vi "StopPull.vi"() -> ()   [LabVIEW 2009]
uses:
  <instrlib>/Newport ESP301/Newport ESP301.lvlib
panel:
  in  "Feedback Filter Settings":T1
  in  "Master Axis":i32
  out "error out":errorcluster
  in  "error in":errorcluster
  out "VISA resource name out":refnum<visa-resource-name>
  in  "VISA resource name":refnum<visa-resource-name>
  in  "Slave Axis":i32
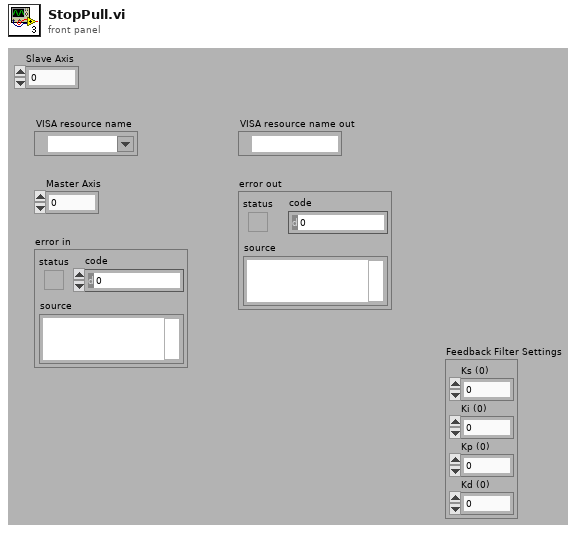
[diagram p1: front panel]
types:
  T1 = cluster{"Ks (0)":dbl, "Ki (0)":dbl, "Kp (0)":dbl, "Kd (0)":dbl}
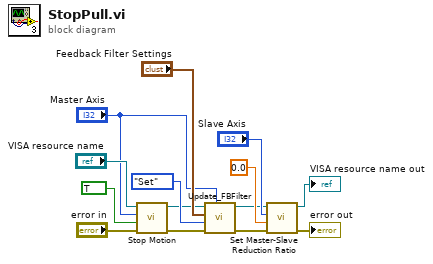
[diagram p0: block diagram]
diagram:
  n1 = call <instrlib>:"Stop Motion.vi"("error in (no error)"="error in", "Stop all axes (F)"=TRUE, "Axis (1)"="Master Axis", "VISA resource name"="VISA resource name") -> ("error out"=w9:errorcluster, "VISA resource name out"=w5:refnum<visa-resource-name>)  [unwired: 2 in]
  n2 = call "Update_FBFilter.vi"("Axis"="Master Axis", "error in (no error)"=w9, "Disable?"=enum16{"Disable", "Set"}."Set", "Feedback Filter Settings"="Feedback Filter Settings", "VISA resource name"=w5) -> ("error out"=w8:errorcluster, "VISA resource name out"=w4:refnum<visa-resource-name>)  [unwired: 5 in]
  n3 = call <instrlib>:"Set Master-Slave Reduction Ratio.vi"("error in (no error)"=w8, "Reduction Ratio (0)"=0.0, "Axis (1)"="Slave Axis", "VISA resource name"=w4) -> ("error out"=→"error out":errorcluster, "VISA resource name out"=→"VISA resource name out":refnum<visa-resource-name>)  [unwired: 2 in]
